vi "Cluster Variant Array to Table Items.vi"(0 "Cluster Variant Array":variant[](array[variant]), 7 "Columns":T1[](array[typedef]), 11 "error in (no error)":errorcluster) -> (4 "Table Items":string[][](array[string]), 8 "rings":i32[][](array[numeric]), 15 "error out":errorcluster)   [LabVIEW 2020]
uses:
  ColumnSpec.ctl
  ColumnType.ctl
  <vilib>/Utility/Data Type/NI_Data Type.lvlib
  KTable.xctl
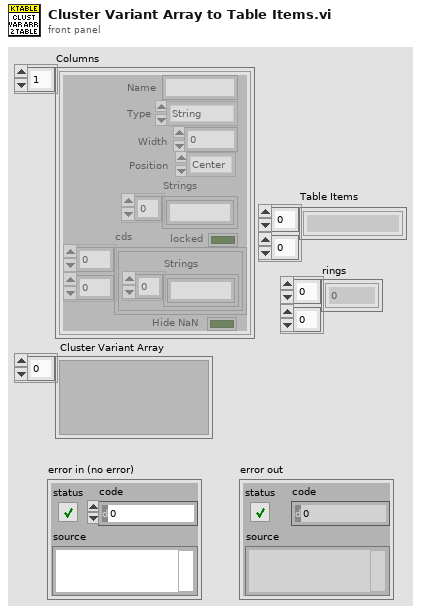
[diagram p1: front panel]
types:
  T1 = typedef "KTable.xctl/ColumnSpec.ctl" = cluster{"Name":string, "Type":T2, "Width":i32, "Strings":string[], "Position":enum16{"Left", "Center", "Right"}, "locked":bool, "cds":cluster{"Strings":string[]}[][], "Hide NaN":bool}
  T2 = typedef "KTable.xctl/ColumnType.ctl" = enum16{"String", "Enum", "Int", "Double", "Boolean", "Ring", "Formula", "Color"}
  T3 = typedef "NI_Data Type.lvlib/Data Type.ctl" = enum8{"Invalid Type", "Void", "I8", "I16", "I32", "I64", "U8", "U16", "U32", "U64", "Single Float", "Double Float", "Extended Float", "Single Complex", "Double Complex", "Extended Complex", "Enum U8", "Enum U16", "Enum U32", "Enum U64", "Single Float With Unit", "Double Float With Unit", "Extended Float With Unit", "Single Complex with Unit", "Double Complex with Unit", "Extended Complex with Unit", "Boolean", "String", "Path", "Picture", "Tag", "Array", "Cluster", "Variant", "LV Variant", "Waveform", "Timestamp", "Digital Waveform", "Digital Data", "ExpressData", "Refnum", "External Data", "VI", "Poly VI", "LabVIEW Class Instance", "Fixed Point", "Set Collection", "Map Collection"}
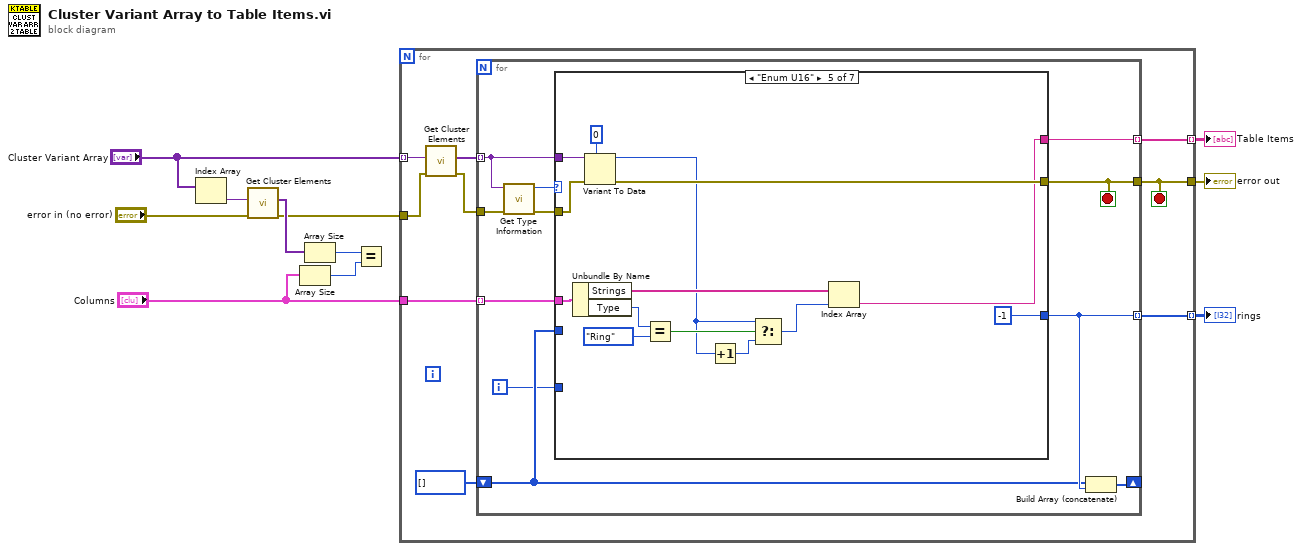
[diagram p0: block diagram]
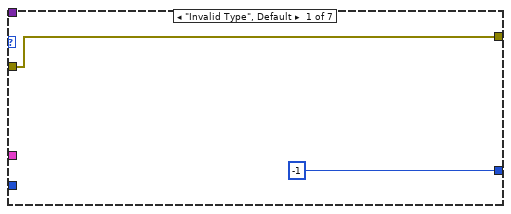
[diagram p2: hidden frame]
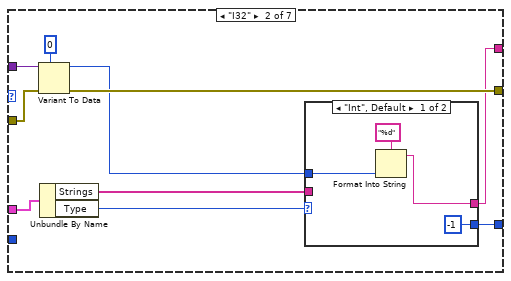
[diagram p3: hidden frame]
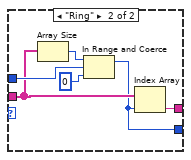
[diagram p4: hidden frame]
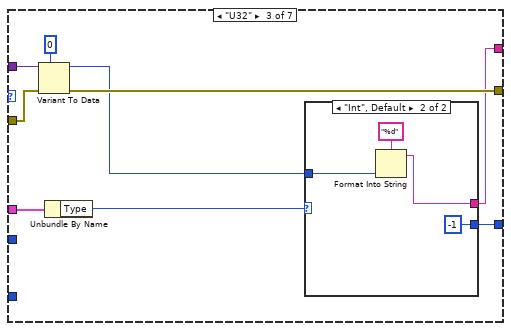
[diagram p5: hidden frame]
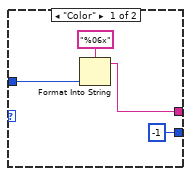
[diagram p6: hidden frame]
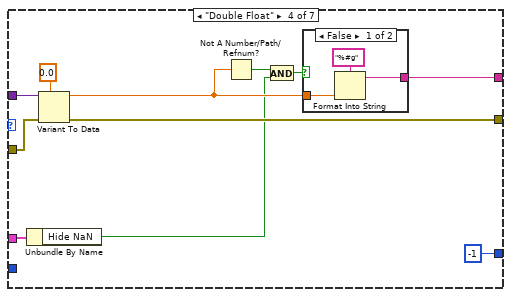
[diagram p7: hidden frame]
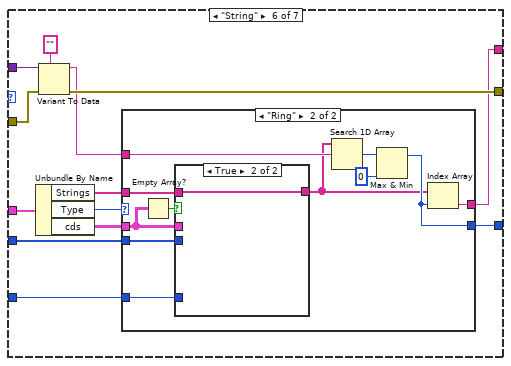
[diagram p9: hidden frame]
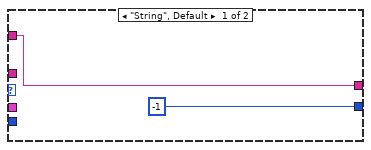
[diagram p10: hidden frame]
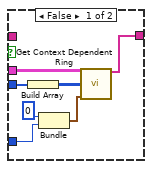
[diagram p11: hidden frame]
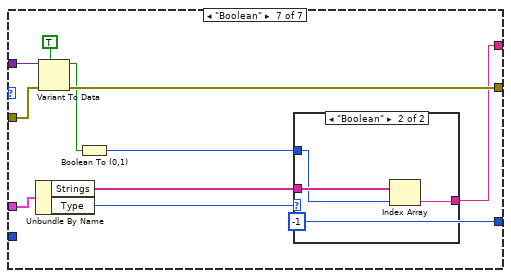
[diagram p12: hidden frame]
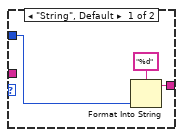
[diagram p13: hidden frame]
diagram:
  n1 = Index Array(array="Cluster Variant Array") -> (element=w11:variant)  [unwired: 1 in]
  n2 = call "Get Cluster Elements.vi"("Error In"="error in (no error)", "Cluster"=w11) -> ("Error Out"=w3:errorcluster, "Cluster Elements"=w10:variant[])  [unwired: 8 in]
  n3 = Array Size(array="Columns") -> (size(s)=w7:i32)
  n4 = Array Size(array=w10) -> (size(s)=w9:i32)
  n5 = Equal?(x=w9, y=w7) -> ()  [unwired: 1 out]
  n6 = for {
    tunnel: "Cluster Variant Array" -> [w20] mode=indexing
    tunnel: "Columns" -> [w19]
    tunnel: [w17] -> w4 mode=indexing
    tunnel: w3 -> [w16]
    tunnel: [w14] -> w2
    tunnel: [w13] -> w1 mode=indexing
    stop <- w14 stop-if-true
    n7 = call "Get Cluster Elements.vi"("Error In"=w16, "Cluster"=w20) -> ("Error Out"=w15:errorcluster, "Cluster Elements"=w18:variant[])  [unwired: 8 in]
    n8 = for {
      tunnel: w19 -> [w25] mode=indexing
      tunnel: w18 -> [w30] mode=indexing
      tunnel: [w29] -> w17 mode=indexing
      tunnel: w15 -> [w28]
      tunnel: [w26] -> w14
      tunnel: [w23] -> w13 mode=indexing
      shift-right: [w24] -> _
      shift-left: i32[] [] -> [w22]
      i -> [w21]
      stop <- w26 stop-if-true
      n9 = call <vilib>:"Get Type Information.vi"("error in (no error)"=w28, "variant"=w30) -> ("error out"=w27:errorcluster, "type"=w31:T3)  [unwired: 5 in, 3 out]
      n10 = case shown="\"Enum U16\"" w31 {
        tunnel: w30 -> [_ w42 w61 w81 w98 w111 w143]
        tunnel: [_ w35 w55 w80 w92 w103 w136] -> w29
        tunnel: w27 -> [w33 w41 w60 w79 w97 w109 w142]
        tunnel: [w33 w40 w59 w78 w96 w108 w141] -> w26
        tunnel: w25 -> [_ w39 w58 w75 w94 w107 w140]
        tunnel: [-1 ("y") w34 w54 -1 ("y") -1 ("y") w102 -1 ("y")] -> w23
        tunnel: w22 -> [_ _ _ _ _ w100 _]
        tunnel: w21 -> [_ _ _ _ _ w99 _]
        frame "Invalid Type", Default {
        }
        frame "I32" {
          n11 = Variant To Data(error in=w41, type=0, Variant=w42) -> (data=w36:i32, error out=w40:errorcluster)
          n12 = Unbundle By Name(w39) -> ("Strings"=w37:string[], "Type"=w38:T2)
          n13 = case shown="\"Int\", Default" w38 {
            tunnel: w37 -> [_ w49]
            tunnel: [w45 w53] -> w35
            tunnel: w36 -> [w46 w51]
            tunnel: [-1 ("y") w48] -> w34
            frame "Int", Default {
              n14 = Format Into String(format string="%d", w46) -> (resulting string=w45:string)  [unwired: 2 in, 1 out]
            }
            frame "Ring" {
              n15 = Array Size(array=w49) -> (size(s)=w50:i32)
              n16 = In Range and Coerce(upper limit=w50, x=w51, lower limit=0 ("y")) -> (coerced(x)=w48:i32)  [unwired: 1 out]
              n17 = Index Array(array=w49, index=w48) -> (element=w53:string)
            }
          }
        }
        frame "U32" {
          n18 = Variant To Data(error in=w60, type=u32 0, Variant=w61) -> (data=w56:u32, error out=w59:errorcluster)
          n19 = Unbundle By Name(w58) -> ("Type"=w57:T2)
          n20 = case shown="\"Int\", Default" w57 {
            tunnel: [w65 w69] -> w55
            tunnel: w56 -> [w63 w67]
            tunnel: [-1 ("y") -1 ("y")] -> w54
            frame "Color" {
              n21 = Format Into String(format string="%06x", w63) -> (resulting string=w65:string)  [unwired: 2 in, 1 out]
            }
            frame "Int", Default {
              n22 = Format Into String(format string="%d", w67) -> (resulting string=w69:string)  [unwired: 2 in, 1 out]
            }
          }
        }
        frame "Double Float" {
          n23 = Unbundle By Name(w75) -> ("Hide NaN"=w71:bool)
          n24 = Variant To Data(error in=w79, type=0.0, Variant=w81) -> (data=w73:dbl, error out=w78:errorcluster)
          n25 = Not A Number/Path/Refnum?(number/path/refnum=w73) -> (NaN/Path/Refnum?=w74:bool)
          n26 = And(x=w74, y=w71) -> (x .and. y?=w72:bool)
          n27 = case shown="False" w72 {
            tunnel: w73 -> [w84 _]
            tunnel: [w82 _] -> w80
            frame False {
              n28 = Format Into String(format string="%#g", w84) -> (resulting string=w82:string)  [unwired: 2 in, 1 out]
            }
            frame True {
            }
          }
        }
        frame "Enum U16" {
          n29 = Unbundle By Name(w94) -> ("Strings"=w93:string[], "Type"=w90:T2)
          n30 = Variant To Data(error in=w97, type=u16 0, Variant=w98) -> (data=w85:u16, error out=w96:errorcluster)
          n31 = Equal?(x=w90, y=ColumnType."Ring") -> (x = y?=w88:bool)
          n32 = Increment(x=w85) -> (x+1=w86:u16)
          n33 = Select(t=w85, s=w88, f=w86) -> (s? t:f=w87:u16)
          n34 = Index Array(array=w93, index=w87) -> (element=w92:string)
        }
        frame "String" {
          n35 = Unbundle By Name(w107) -> ("Strings"=w104:string[], "Type"=w106:T2, "cds"=w101:cluster{"Strings":string[]}[][])
          n36 = Variant To Data(error in=w109, type="", Variant=w111) -> (data=w105:string, error out=w108:errorcluster)
          n37 = case shown="\"Ring\"" w106 {
            tunnel: w105 -> [w113 w124]
            tunnel: w104 -> [_ w119]
            tunnel: [w113 w121] -> w103
            tunnel: [-1 w120] -> w102
            tunnel: w101 -> [_ w116]
            tunnel: w100 -> [_ w115]
            tunnel: w99 -> [_ w114]
            frame "String", Default {
            }
            frame "Ring" {
              n38 = Empty Array?(array=w116) -> (empty?=w118:bool)
              n39 = case shown="True" w118 {
                tunnel: w119 -> [_ w132]
                tunnel: [w130 w132] -> w117
                tunnel: w116 -> [w131 _]
                tunnel: w115 -> [w129 _]
                tunnel: w114 -> [w125 _]
                frame False {
                  n40 = Build Array(w129) -> (w128:i32[][])
                  n41 = Bundle(0, w125) -> (w126:cluster{i32, i32})  [unwired: 1 in]
                  n42 = call "Get Context Dependent Ring.vi"("cds"=w131, "rings"=w128, "Cell Position"=w126) -> ("Strings"=w130:string[])  [unwired: 12 in]
                }
                frame True {
                }
              }
              n43 = Search 1D Array(1D array=w117, element=w124) -> (index of element=w123:i32)  [unwired: 1 in]
              n44 = Max & Min(x=w123, y=0) -> (max(x,y)=w120:i32)  [unwired: 1 out]
              n45 = Index Array(array=w117, index=w120) -> (element=w121:string)
            }
          }
        }
        frame "Boolean" {
          n46 = Unbundle By Name(w140) -> ("Strings"=w137:string[], "Type"=w139:T2)
          n47 = Variant To Data(error in=w142, type=TRUE, Variant=w143) -> (data=w138:bool, error out=w141:errorcluster)
          n48 = Boolean To (0,1)(Boolean=w138) -> (0, 1=w134:i16)
          n49 = case shown="\"Boolean\"" w139 {
            tunnel: w134 -> [w144 w148]
            tunnel: w137 -> [_ w149]
            tunnel: [w146 w147] -> w136
            frame "String", Default {
              n50 = Format Into String(format string="%d", w144) -> (resulting string=w146:string)  [unwired: 2 in, 1 out]
            }
            frame "Boolean" {
              n51 = Index Array(array=w149, index=w148) -> (element=w147:string)
            }
          }
        }
      }
      n52 = Build Array (concatenate)(w22, w23) -> (w24:i32[])
    }
  }
  "error out" <- w2
  "Table Items" <- w4
  "rings" <- w1
